vi "CheckButtoneTrue.vi"(10 "IN":bool) -> (3 "OUT":bool)   [LabVIEW 2014, in "LibraryGcode.lvlib"]
uses:
  LibraryGcode.lvlib
  variableGlobal/StartAutoandGcode.vi
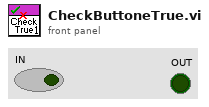
[diagram p1: front panel]
types:
  T1 = typedef "stateModeDevice.ctl" = enum16{"Auto", "Menu", "WaitAutoFinish", "Config", "initAuto"}
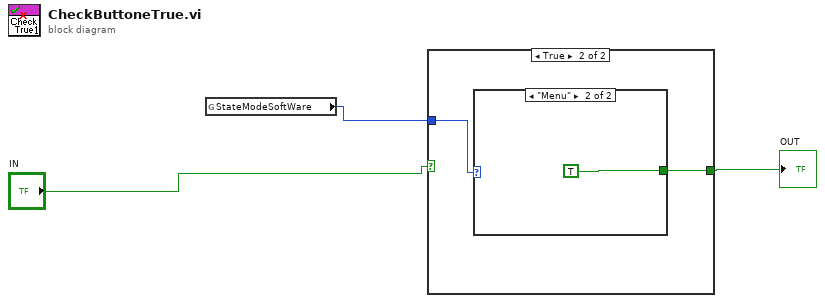
[diagram p0: block diagram]
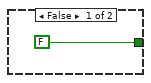
[diagram p2: hidden frame]
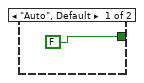
[diagram p3: hidden frame]
diagram:
  n1 = global read "StartAutoandGcode.vi" "StateModeSoftWare"() -> (w1:T1)
  n2 = case shown="True" "IN" {
    tunnel: [FALSE ("OUT") w6] -> w3
    tunnel: w1 -> [_ w5]
    frame False {
    }
    frame True {
      n3 = case shown="\"Menu\"" w5 {
        tunnel: [FALSE ("OUT") TRUE ("OUT")] -> w6
        frame "Auto", Default {
        }
        frame "Menu" {
        }
      }
    }
  }
  "OUT" <- w3
